vi "newFile.vi"(8 "error in (no error)":errorcluster, 11 "reference in":refnum<class "File Controller.lvclass">) -> (0 "error out":errorcluster, 3 "reference out":refnum<class "File Controller.lvclass">)   [LabVIEW 2015, in "File Controller.lvclass"]
uses:
  File Controller.lvclass
  APP/excelFile_class/excelFile.lvclass
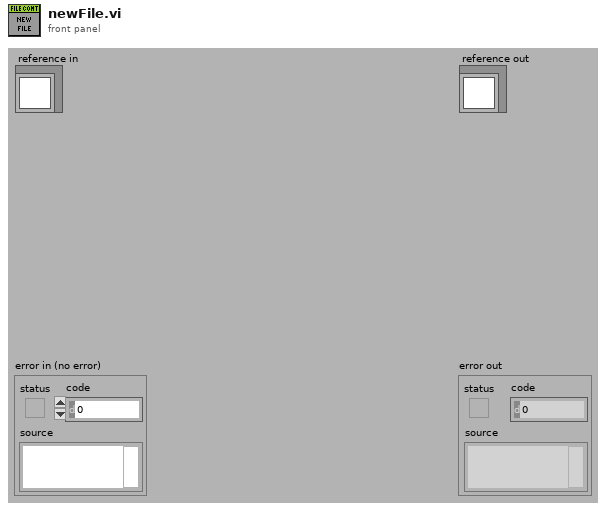
[diagram p1: front panel]
types:
  T1 = typedef "File Controller.lvclass/ObjectAttributesRef.ctl" = refnum<data-value>
  T2 = typedef "File Controller.lvclass/ObjectAttributes.ctl" = cluster{"MyAttribute":dbl, "file_path":path, "file_type":T3, "data":string[][][], "excel_file_ref":refnum<class "excelFile.lvclass">, "sheetName":string[], "subject_refs":refnum<class "subject.lvclass">[], "temp_data":string[][][]}
  T3 = typedef "excelFile.lvclass/fileType.ctl" = enum16{"database", "CosmedTest"}
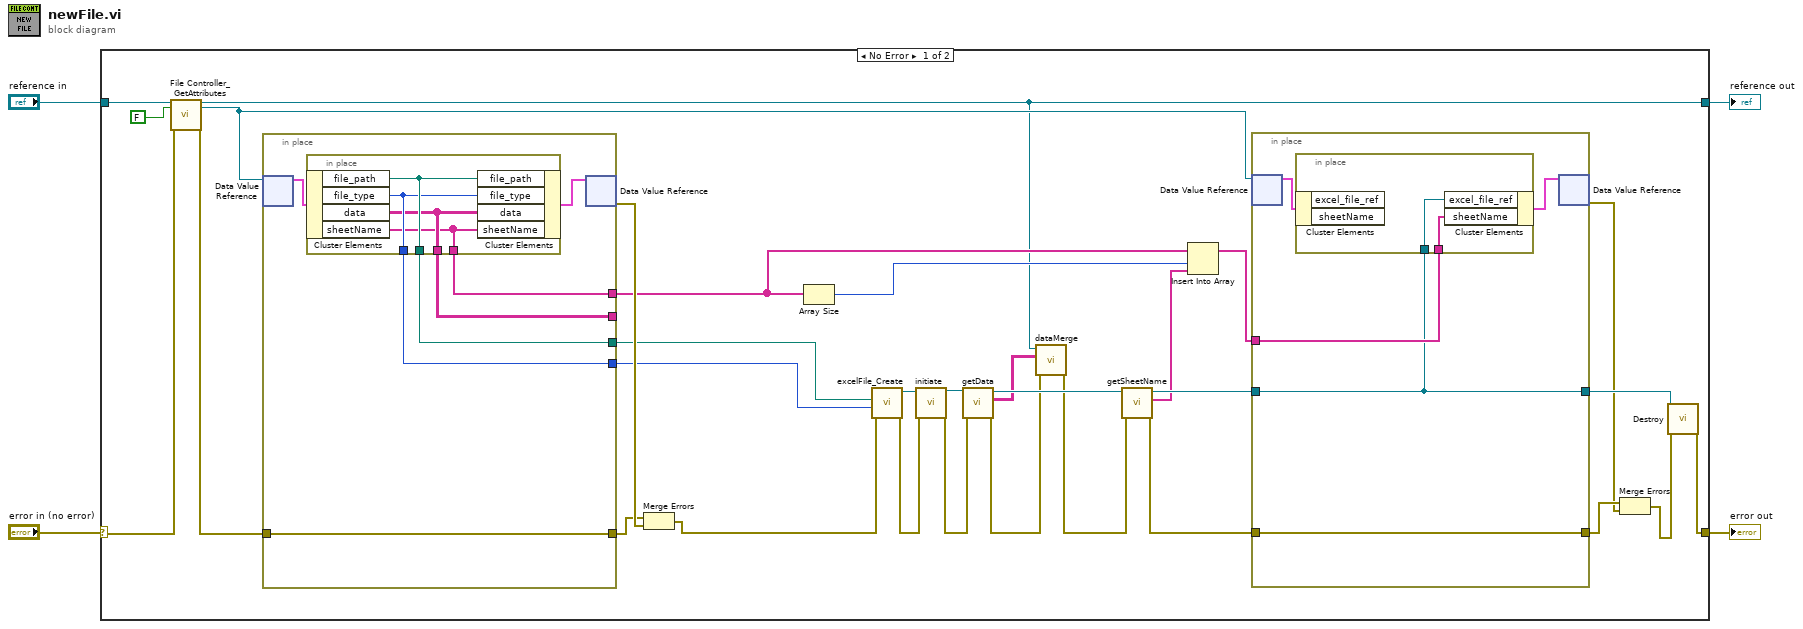
[diagram p0: block diagram]
diagram:
  n1 = case shown="No Error" "error in (no error)" {
    selector: "error in (no error)" -> [w30 w54]
    tunnel: [w12 w54] -> w3
    tunnel: [w5 w53] -> w1
    tunnel: "reference in" -> [w32 w53]
    frame No Error {
      n2 = call "File Controller_GetAttributes.vi"("reference in"=w32, "return data? (T)"=FALSE, "error in (no error)"=w30) -> ("reference out"=w5:refnum<class "File Controller.lvclass">, "attributes ref"=w25:T1, "error out"=w29:errorcluster)  [unwired: 13 in, 1 out]
      n3 = in-place {
        in-place-border: w29 -> [w46]
        in-place-border: [w46] -> w33
        in-place-border: [w45] -> w28
        in-place-border: [w44] -> w27
        in-place-border: [w43] -> _
        in-place-border: [w42] -> w17
        n4 = in-place-dvr #1(w25) -> (w47:T2)  [unwired: 1 out]
        n5 = in-place {
          in-place-border: [w52] -> w45
          in-place-border: [w51] -> w44
          in-place-border: [w50] -> w43
          in-place-border: [w49] -> w42
          n6 = in-place-cluster #2(w47) -> ("file_path"=w52:path, "file_type"=w51:T3, "data"=w50:string[][][], "sheetName"=w49:string[])
          n7 = in-place-cluster #2("file_path"=w52, "file_type"=w51, "data"=w50, "sheetName"=w49) -> (w48:T2)
        }
        n8 = in-place-dvr #1(w48) -> (w34:errorcluster)  [unwired: 1 out]
      }
      n9 = Merge Errors(w33, w34) -> (w26:errorcluster)
      n10 = Array Size(array=w17) -> (size(s)=w16:i32)
      n11 = call "excelFile_Create.vi"("error in (no error)"=w26, "fileType"=w27, "Path"=w28) -> ("error out"=w23:errorcluster, "reference out"=w24:refnum<class "excelFile.lvclass">)  [unwired: 7 in]
      n12 = call-dynamic "initiate.vi"("reference in"=w24, "error in (no error)"=w23) -> ("reference out"=w22:refnum<class "excelFile.lvclass">, "error out"=w21:errorcluster)  [unwired: 16 in]
      n13 = call "getData.vi"("error in (no error)"=w21, "reference in"=w22) -> ("error out"=w7:errorcluster, "data"=w8:string[][][], "reference out"=w20:refnum<class "excelFile.lvclass">)  [unwired: 7 in]
      n14 = call "dataMerge.vi"("error in (no error)"=w7, "data"=w8, "reference in"=w5) -> ("error out"=w6:errorcluster)  [unwired: 7 in, 1 out]
      n15 = call "getSheetName.vi"("error in (no error)"=w6, "reference in"=w20) -> ("error out"=w19:errorcluster, "sheetName"=w15:string[], "reference out"=w18:refnum<class "excelFile.lvclass">)  [unwired: 7 in]
      n16 = Insert Into Array(array=w17, index=w16, new element=w15) -> (w14:string[])
      n17 = in-place {
        in-place-border: w19 -> [w37]
        in-place-border: [w37] -> w11
        in-place-border: w14 -> [w36]
        in-place-border: w18 -> [w35]
        in-place-border: [w35] -> w13
        n18 = in-place-dvr #3(w25) -> (w38:T2)  [unwired: 1 out]
        n19 = in-place {
          in-place-border: w36 -> [w41]
          in-place-border: w35 -> [w40]
          n20 = in-place-cluster #4(w38) -> ()  [unwired: 2 out]
          n21 = in-place-cluster #4("excel_file_ref"=w40, "sheetName"=w41) -> (w39:T2)
        }
        n22 = in-place-dvr #3(w39) -> (w9:errorcluster)  [unwired: 1 out]
      }
      n23 = Merge Errors(w11, w9) -> (w10:errorcluster)
      n24 = call-dynamic "Destroy.vi"("reference in"=w13, "error in (no error)"=w10) -> ("error out"=w12:errorcluster)  [unwired: 16 in, 1 out]
    }
    frame Error {
    }
  }
  "error out" <- w3
  "reference out" <- w1
